vi "punto1.vi"() -> ()   [LabVIEW 2018]
panel:
  out "Sensor De Temperatura °c":dbl(slide) scale=0.0..100.0
  in  "Selector":bool
  in  "Rata (5°c/seg)":dbl(knob)=1.0 scale=1.0..10.0
  # "Incrementar"
  # "Decrementar"
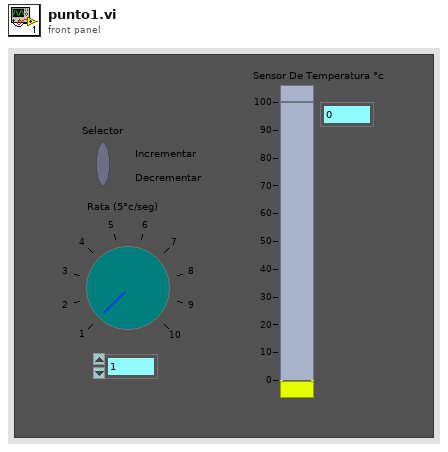
[diagram p1: front panel]
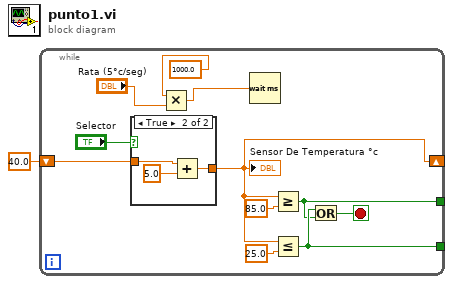
[diagram p0: block diagram]
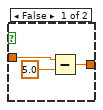
[diagram p2: hidden frame]
diagram:
  n1 = while {
    shift-right: [w8] -> _
    shift-left: 40.0 -> [w12]
    tunnel: [w5] -> _
    tunnel: [w6] -> _
    stop <- w7 stop-if-true
    n2 = case shown="True" "Selector" {
      tunnel: [w15 w18] -> w8
      tunnel: w12 -> [w14 w17]
      frame False {
        n3 = Subtract(x=w14, y=5.0) -> (x-y=w15:dbl)
      }
      frame True {
        n4 = Add(x=w17, y=5.0) -> (x+y=w18:dbl)
      }
    }
    "Sensor De Temperatura °c" <- w8
    n5 = Multiply(x=1000.0, y="Rata (5°c/seg)") -> (x*y=w4:dbl)
    n6 = Wait (ms)(milliseconds to wait=w4) -> ()  [unwired: 1 out]
    n7 = Greater Or Equal?(x=w8, y=85.0) -> (x >= y?=w5:bool)
    n8 = Less Or Equal?(x=w8, y=25.0) -> (x <= y?=w6:bool)
    n9 = Or(x=w6, y=w5) -> (x .or. y?=w7:bool)
  }
